vi "Refresh Info.vi"(8 "error in (no error)":errorcluster, 11 "Device in":refnum<class "Device.lvclass">) -> (0 "error out":errorcluster, 3 "Device out":refnum<class "Device.lvclass">)   [LabVIEW 2020, in "PicoG-Core.lvlib" / "Device.lvclass"]
uses:
  Device.lvclass
  Device.lvclass/Device.ctl
  DeployResource/DeployResource.lvclass
  PicoG-Core.lvlib
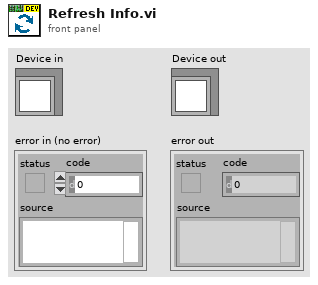
[diagram p1: front panel]
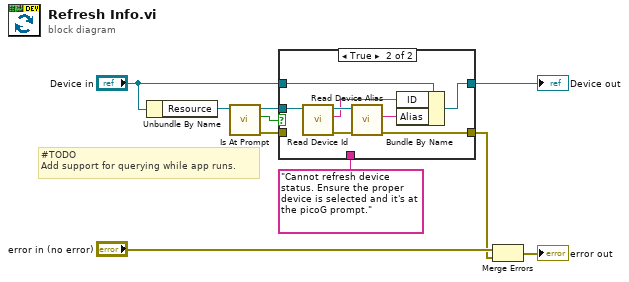
[diagram p0: block diagram]
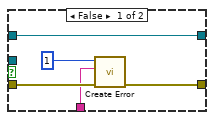
[diagram p2: hidden frame]
diagram:
  # "#TODO\nAdd support for querying while app runs."
  n1 = Unbundle By Name("Device in") -> ("Resource"=w9:refnum<class "DeployResource.lvclass">)
  n2 = call-dynamic "Is At Prompt.vi"("DeployResource in"=w9) -> ("error out"=w6:errorcluster, "At Prompt?"=w8:bool, "DeployResource out"=w7:refnum<class "DeployResource.lvclass">)  [unwired: 7 in, 1 out]
  n3 = case shown="True" w8 {
    tunnel: w7 -> [_ w22]
    tunnel: w6 -> [w15 _]
    tunnel: "Cannot refresh device status. Ensure the proper device is selected and it's at the picoG prompt." ("Message (\"\")") -> [w14 _]
    tunnel: [w12 w19] -> w1
    tunnel: "Device in" -> [w11 w23]
    tunnel: [w11 w18] -> w3
    frame False {
      n4 = call "Create Error.vi"("error in (no error)"=w15, "Message (\"\")"=w14, "Code"=1) -> ("error out"=w12:errorcluster)  [unwired: 8 in]
    }
    frame True {
      n5 = call "Read Device Id.vi"("Resource in"=w22) -> ("error out"=w20:errorcluster, "Id"=w17:string, "Resource out"=w21:refnum<class "DeployResource.lvclass">)  [unwired: 8 in]
      n6 = call "Read Device Alias.vi"("error in (no error)"=w20, "Resource in"=w21) -> ("error out"=w19:errorcluster, "Alias"=w16:string)  [unwired: 7 in, 1 out]
      n7 = Bundle By Name(cluster=w23, "ID"=w17, "Alias"=w16) -> (w18:refnum<class "Device.lvclass">)
    }
  }
  "Device out" <- w3
  n8 = Merge Errors("error in (no error)", w1) -> (→"error out":errorcluster)
